vi "RampOrLin.vi"() -> ()   [LabVIEW 2011]
panel:
  in  "Kinetice chooser":enum32{"Linear", "Stepwise"}(radio)
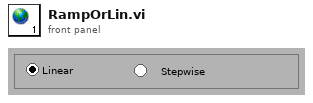
[diagram p1: front panel]
diagram:
